vi "GetTypeDefs.vi"(0 "ClassReader in":refnum<class "ClassReader.lvclass">, 5 "error in (no error)":errorcluster) -> (14 "ClassReader out":refnum<class "ClassReader.lvclass">, 15 "TypeDefs":T1[](array[typedef]), 19 "error out":errorcluster)   [LabVIEW 2020, in "ClassReader.lvclass"]
uses:
  <resource>/Framework/Providers/Open_GDS/ClassProviders/Provider_BaseClassInterface/ClassReader_class/ClassReader.lvclass
  <resource>/Framework/Providers/Open_GDS/UML/ReversedEngineering/ReversedEngineering TypeDefType.ctl
  <resource>/Framework/Providers/Open_GDS/UML/ReversedEngineering/ReversedEngineering AttributeInfoType.ctl
  <resource>/Framework/Providers/Open_GDS/ClassProviders/Common/CommonVIs/CommonVIs_AttributeDataType.ctl
  <resource>/Framework/Providers/Open_GDS/UML/UMLEditor/UMLEditor_VisibilityType.ctl
  <resource>/Framework/Providers/Open_GDS/ClassProviders/Provider_BaseClassInterface/ClassReader_class/ClassReader.lvclass/ClassReader.ctl
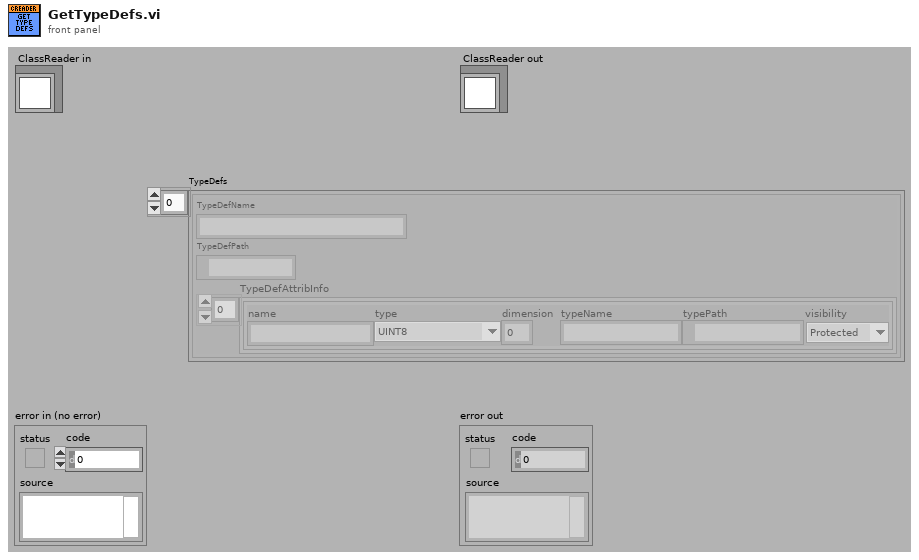
[diagram p1: front panel]
types:
  T1 = typedef "ReversedEngineering TypeDefType.ctl" = cluster{"TypeDefName":string, "TypeDefPath":path, "TypeDefAttribInfo":T2[]}
  T2 = typedef "ReversedEngineering AttributeInfoType.ctl" = cluster{"name":string, "type":T3, "dimension":i32, "typeName":string, "typePath":path, "visibility":T4}
  T3 = typedef "CommonVIs_AttributeDataType.ctl" = enum16{"UINT8", "INT8", "UINT16", "INT16", "UINT32", "INT32", "UINT64", "INT64", "SGL", "DBL", "EXT", "CSG", "CDB", "CXT", "TimeStamp", "STRING", "PATH", "BOOL", "ENUM", "RefNum", "VIRefNum", "LabVIEW Class", "Cluster", "Variant", "TypeDef", "Waveform", "LabVIEW Object", "Other", "void", "Set", "Map"}
  T4 = typedef "UMLEditor_VisibilityType.ctl" = enum16{"Public", "Private", "Protected"}
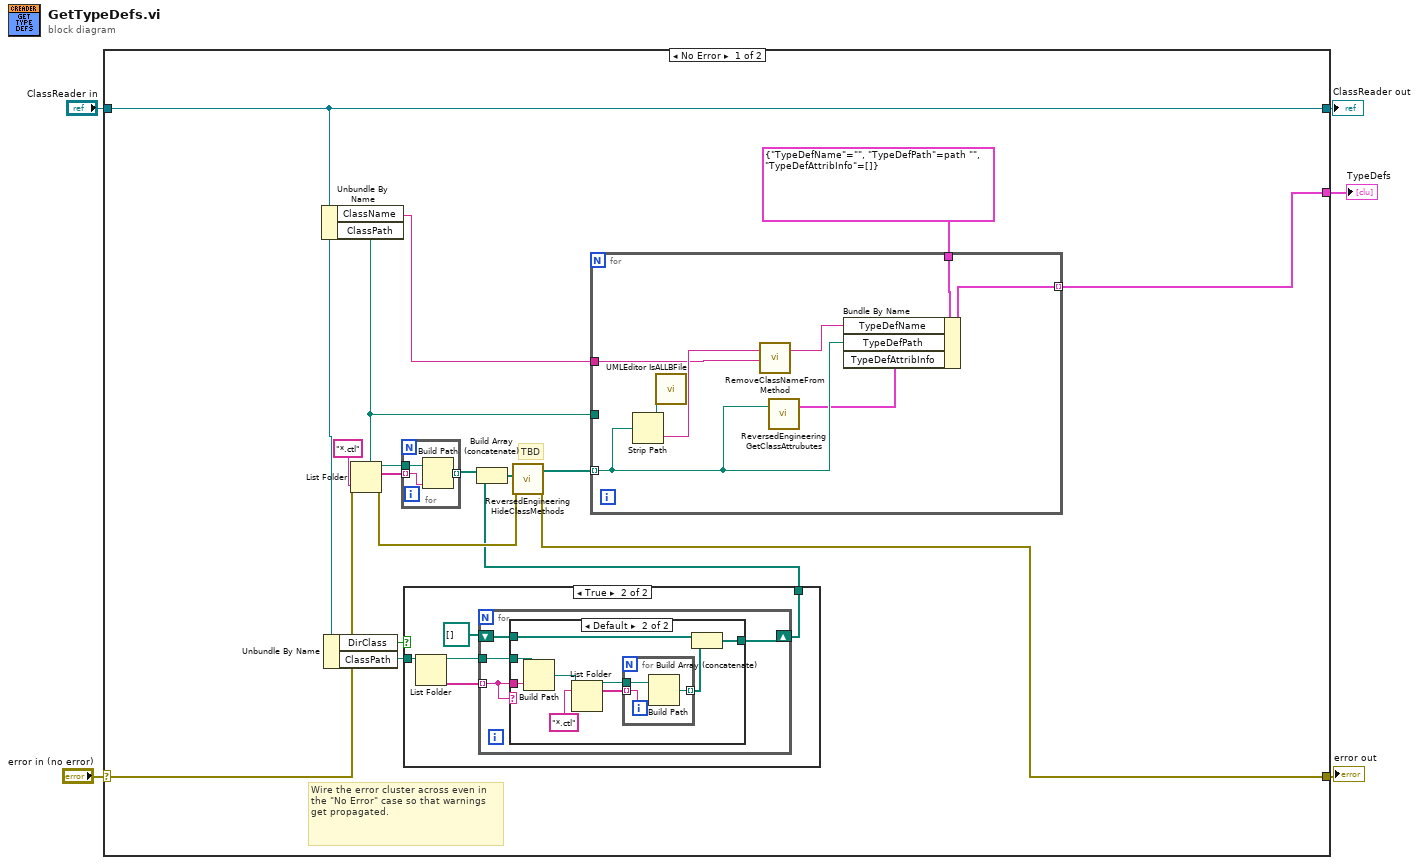
[diagram p0: block diagram]
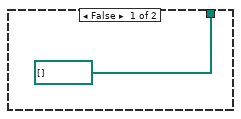
[diagram p2: hidden frame]
diagram:
  n1 = case shown="No Error" "error in (no error)" {
    selector: "error in (no error)" -> [w10 w58]
    tunnel: [w8 w58] -> w4
    tunnel: [w9 w57] -> w2
    tunnel: "ClassReader in" -> [w9 w57]
    tunnel: [w6 _] -> w1
    frame No Error {
      # "TBD"
      # "Wire the error cluster across even in the \"No Error\" case so that warnings get propagated."
      n2 = Unbundle By Name(w9) -> ("ClassName"=w14:string, "ClassPath"=w11:path)
      n3 = Unbundle By Name(w9) -> ("DirClass"=w16:bool, "ClassPath"=w15:path)
      n4 = List Folder(path=w11, pattern="*.ctl", error in=w10) -> (path out=w22:path, filenames=w21:string[], error out=w18:errorcluster)  [unwired: 1 in, 1 out]
      n5 = for {
        tunnel: w22 -> [w56]
        tunnel: w21 -> [w54] mode=indexing
        tunnel: [w55] -> w20 mode=indexing
        n6 = Build Path(base path=w56, name or relative path=w54) -> (appended path=w55:path)
      }
      n7 = case shown="True" w16 {
        tunnel: w15 -> [_ w28]
        tunnel: [path[] [] w25] -> w13
        frame False {
        }
        frame True {
          n8 = List Folder(path=w28) -> (path out=w27:path, folder names=w26:string[])  [unwired: 3 in, 2 out]
          n9 = for {
            tunnel: w27 -> [w32]
            tunnel: w26 -> [w29] mode=indexing
            shift-right: [w30] -> w25
            shift-left: path[] [] -> [w31]
            n10 = case shown="Default" w29 {
              tunnel: w32 -> [_ w39]
              tunnel: w29 -> [_ w38]
              tunnel: w31 -> [w33 w36]
              tunnel: [w33 w35] -> w30
              frame "Example", "Examples", "Test" {
              }
              frame Default {
                n11 = Build Path(base path=w39, name or relative path=w38) -> (appended path=w37:path)
                n12 = List Folder(path=w37, pattern="*.ctl") -> (path out=w41:path, filenames=w42:string[])  [unwired: 2 in, 2 out]
                n13 = for {
                  tunnel: w41 -> [w45]
                  tunnel: w42 -> [w43] mode=indexing
                  tunnel: [w44] -> w34 mode=indexing
                  n14 = Build Path(base path=w45, name or relative path=w43) -> (appended path=w44:path)
                }
                n15 = Build Array (concatenate)(w36, w34) -> (w35:path[])
              }
            }
          }
        }
      }
      n16 = Build Array (concatenate)(w20, w13) -> (w12:path[])
      n17 = call <resource>:"ReversedEngineering HideClassMethods.vi"("Item Paths"=w12, "error in (no error)"=w18) -> ("Item Paths filtered"=w19:path[], "error out"=w8:errorcluster)  [unwired: 16 in]
      n18 = for {
        tunnel: w19 -> [w47] mode=indexing
        tunnel: w14 -> [w51]
        tunnel: w11 -> [_]
        tunnel: [w48] -> w6 mode=indexing
        tunnel: T1 {"TypeDefName"="", "TypeDefPath"=path "", "TypeDefAttribInfo"=[]} ("TypeDef") -> [w50]
        n19 = Strip Path(path=w47) -> (stripped path=w53:path, name=w52:string)
        n20 = call <resource>:"UMLEditor IsALLBFile.vi"("path"=w53) -> ()  [unwired: 1 out]
        n21 = call <resource>:"RemoveClassNameFromMethod.vi"("MethodVINameIn"=w52, "ClassName"=w51) -> ("MethodVINameOut"=w49:string)  [unwired: 17 in]
        n22 = call <resource>:"ReversedEngineering GetClassAttrubutes.vi"("Path(CtrlRenumf used if Path is empty)"=w47) -> ("attributeInfo"=w46:T2[])  [unwired: 16 in, 2 out]
        n23 = Bundle By Name(cluster=w50, "TypeDefName"=w49, "TypeDefPath"=w47, "TypeDefAttribInfo"=w46) -> (w48:T1)
      }
    }
    frame Error {
    }
  }
  "error out" <- w4
  "ClassReader out" <- w2
  "TypeDefs" <- w1
